vi "Read Channel Map.vi"(8 "error in (no error)":errorcluster, 11 "Zenoh in":refnum<class "Zenoh.lvclass">) -> (0 "error out":errorcluster, 2 "Channel Map":map{string, T1}(c390), 3 "Zenoh out":refnum<class "Zenoh.lvclass">)   [LabVIEW 2021, in "Zenoh.lvclass"]
uses:
  Zenoh.lvclass
  Zenoh.lvclass/Zenoh.ctl
  typedef/Channel Info.ctl
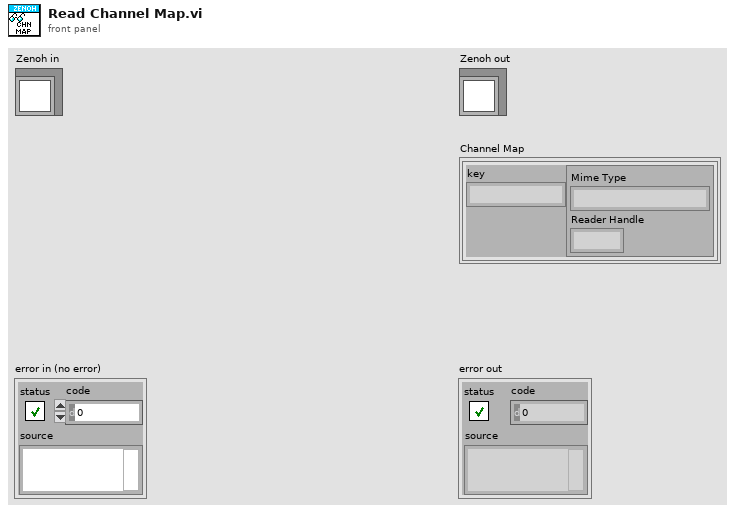
[diagram p1: front panel]
types:
  T1 = typedef "Zenoh.lvclass/Channel Info.ctl" = cluster{"Mime Type":string, "Reader Handle":u64}
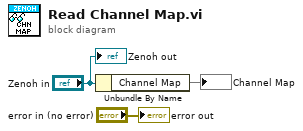
[diagram p0: block diagram]
diagram:
  n1 = Unbundle By Name("Zenoh in") -> ("Channel Map"=→"Channel Map":map{string, T1})
  "error out" <- "error in (no error)"
  "Zenoh out" <- "Zenoh in"
